vi "SystemController.GetImage.vi"(8 "error in (no error)":errorcluster, 10 "index (0 = most recent)":i32, 11 "SystemController":refnum<class "SystemController.lvclass">) -> (0 "error out":errorcluster, 2 "Image":T1, 3 "SystemController out":refnum<class "SystemController.lvclass">)   [LabVIEW 2017, in "SystemController.lvclass"]
doc: "---------------------------------------------------------------\nJKI State Machine Objects™\nhttp://jki.net/state-machine-objects/\nCopyright (C) 2005-2015, JKI <info@jki.net>\nALL RIGHTS RESERVEDJKI State Machine Objects (SMO) 1.0.0.5\nJKI - JKI\nCopyright (c) 2016, JKI"
uses:
  SystemController.lvclass
  <vilib>/vision/Image Controls.llb/IMAQ Image.ctl
  SystemController.lvclass/SystemController.ctl
panel:
  # "For instructions on how to use the JKI State Machine Objects, examples and video tutorials, visit:\nhttp://jki.net/state-machine-objects/\n\nJKI State Machine Objects™\nhttp://jki.net/state-machine-objects/\nCopyright (C) 2005-2015, JKI <info@jki.net>\nALL RIGHTS RESERVED"
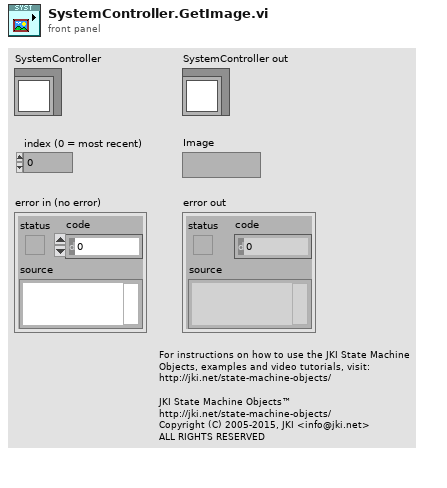
[diagram p1: front panel]
types:
  T1 = typedef "IMAQ Image.ctl" = refnum<image>
  T2 = typedef "SystemController.lvclass/PrivateData--Ref.ctl" = refnum<data-value>
  T3 = typedef "SystemController.lvclass/PrivateData--Cluster.ctl" = cluster{"Configuration":T4, "Dependencies":T8, "Public Events":T9, "Processed Image Buffer":T1[]}
  T4 = typedef "SystemController.lvclass/Configuration--Cluster.ctl" = cluster{"Camera":T5, "Find Eyes":bool, "Acquisition Rate (ms)":i32, "Image Buffer Length":i32}
  T5 = typedef "SystemController.lvclass/CameraConfig--Cluster.ctl" = cluster{"Simulate Camera":bool, "IMAQ Camera":T6, "Simulated Image Folder":path}
  T6 = typedef "Camera_IMAQdx.lvclass/Configuration--Cluster.ctl" = cluster{"Camera Interface Name":string, "Number of Buffers":u32, "Image Name":string, "Image Type":T7}
  T7 = typedef "Image Type" = u32
  T8 = typedef "SystemController.lvclass/Dependencies--Cluster.ctl" = cluster{"Camera":refnum<class "Camera.lvclass">, "ImageFacialDetection":refnum<class "ImageFacialDetection.lvclass">}
  T9 = typedef "SystemController.lvclass/PublicEvents--Cluster.ctl" = cluster{"UIClosed":refnum<user-event>}
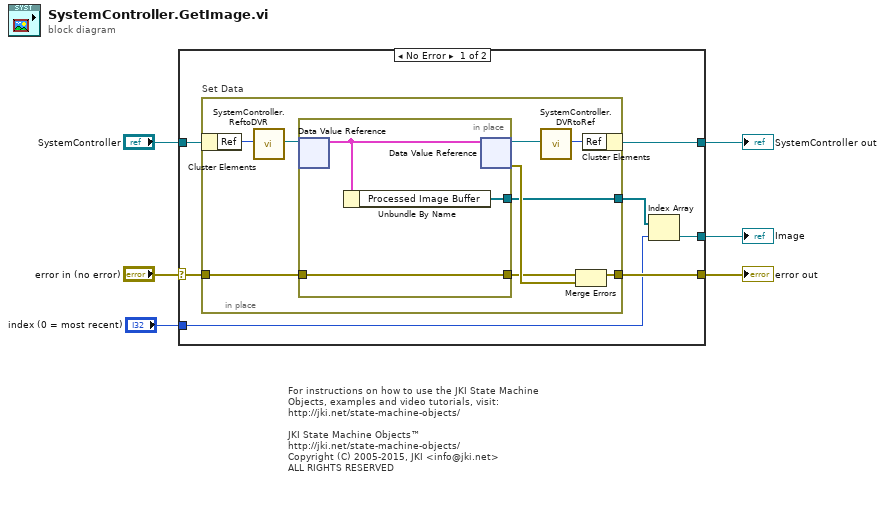
[diagram p0: block diagram]
diagram:
  # "For instructions on how to use the JKI State Machine Objects, examples and video tutorials, visit:\nhttp://jki.net/state-machine-objects/\n\nJKI State Machine Objects™\nhttp://jki.net/state-machine-objects/\nCopyright (C) 2005-2015, JKI <info@jki.net>\nALL RIGHTS RESERVED"
  n1 = case shown="No Error" "error in (no error)" {
    selector: "error in (no error)" -> [w12 w26]
    tunnel: "SystemController" -> [w13 w27]
    tunnel: [w11 w26] -> w5
    tunnel: [w10 w27] -> w4
    tunnel: [w8 _] -> w2
    tunnel: "index (0 = most recent)" -> [w9 _]
    frame No Error {
      n2 = in-place "Set Data" {
        in-place-border: w12 -> [w22]
        in-place-border: [w19] -> w11
        in-place-border: [w14] -> w7
        n3 = in-place-cluster #1(w13) -> ("Ref"=w18:u32)
        n4 = call "SystemController.ReftoDVR.vi"("Ref"=w18) -> ("Ref"=w17:T2)  [unwired: 10 in]
        n5 = in-place {
          in-place-border: w22 -> [w25]
          in-place-border: [w25] -> w20
          in-place-border: [w23] -> w14
          n6 = in-place-dvr #2(w17) -> (w24:T3)  [unwired: 1 out]
          n7 = Unbundle By Name(w24) -> ("Processed Image Buffer"=w23:T1[])
          n8 = in-place-dvr #2(w24) -> (w16:T2, w21:errorcluster)
        }
        n9 = call "SystemController.DVRtoRef.vi"("Ref"=w16) -> ("Ref"=w15:u32)  [unwired: 10 in]
        n10 = Merge Errors(w20, w21) -> (w19:errorcluster)
        n11 = in-place-cluster #1("Ref"=w15) -> (w10:refnum<class "SystemController.lvclass">)
      }
      n12 = Index Array(array=w7, index=w9) -> (element=w8:T1)
    }
    frame Error {
    }
  }
  "error out" <- w5
  "SystemController out" <- w4
  "Image" <- w2
